vi "SPI Send Receive.vi"(7 "Chip Select DIO Pin":u8, 8 "Error In":errorcluster, 9 "Word Size (Bytes)":u8, 10 "SPI Data":u8[](array[numeric]), 11 "Arduino Resource":T1={"COM Port"="COM4", "Board Type"=enum."ChipKit uC32", "Connection Type"=enum."USB / Serial", "Baud Rate (115200)"=15, "Bytes Per Packet (15)"=15}) -> (0 "Error Out":errorcluster, 2 "SPI Data":u8[](array[numeric]), 3 "Arduino Resource":T1={"COM Port"="COM4", "Board Type"=enum."ChipKit uC32", "Connection Type"=enum."USB / Serial", "Baud Rate (115200)"=15, "Bytes Per Packet (15)"=15})   [LabVIEW 2011, in "LabVIEW Interface for ChipKit.lvlib"]
doc: "Send / Receive data bytes on the SPI bus. You must initialize the bus before you can use this VI to send / receive data."
uses:
  LabVIEW Interface for ChipKit.lvlib
  Private/Type Defs/Chipkit Resource.ctl
  Private/Type Defs/Board Type.ctl
  Private/Type Defs/Connection Type.ctl
  Private/Type Defs/Command.ctl
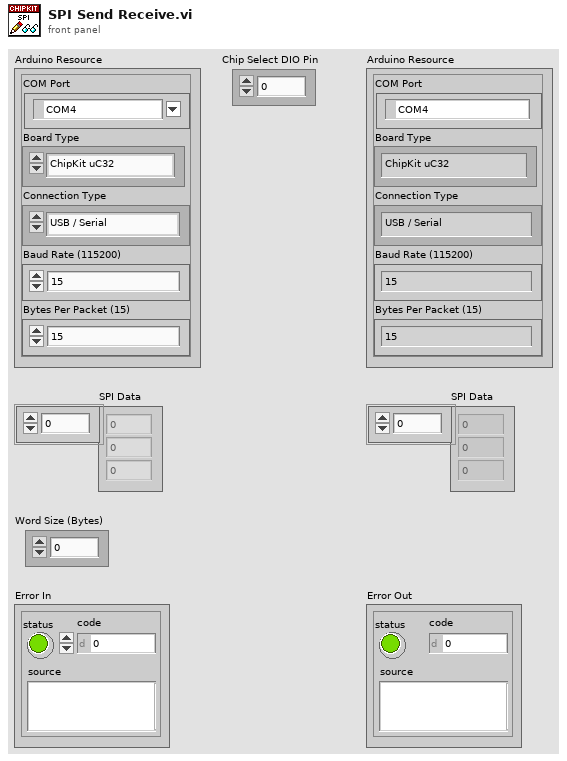
[diagram p1: front panel]
types:
  T1 = typedef "LabVIEW Interface for ChipKit.lvlib/Chipkit Resource.ctl" = cluster{"COM Port":refnum<visa-resource-name>, "Board Type":T2, "Connection Type":T3, "Baud Rate (115200)":u32, "Bytes Per Packet (15)":u32}
  T2 = typedef "LabVIEW Interface for ChipKit.lvlib/Board Type.ctl" = enum16{"ChipKit uC32", "ChipKit Uno32", "ChipKit Max32"}
  T3 = typedef "LabVIEW Interface for ChipKit.lvlib/Connection Type.ctl" = enum8{"USB / Serial", "XBEE", "BlueSmirf (Bluetooth)"}
  T4 = typedef "LabVIEW Interface for ChipKit.lvlib/Command.ctl" = enum8{"setArduinoMode", "flushSerial", "setPinMode", "digitalWritePin", "digitalWritePort", "tone", "digitalReadPin", "digitalReadPort", "analogReadPin", "analogReadPort", "pwmWritePin", "pwmWritePort", "sevenSegment_Configure", "sevenSegment_Write", "I2C Init", "I2C Write", "I2C Read", "SPI Init", "SPI Set Bit Order", "SPI Set Clock Divider", "SPI Set Data Mode", "SPI Send / Receive", "SPI Close", "Servo Set Num Servos", "Servo Config Servo", "Servo Write Angle", "Servo Read Angle", "Servo Write Pulse Width", "Servo Read Pulse Width", "Servo Detach", "LCD Init", "LCD Set Size", "LCD Set Cursor Mode", "LCD Clear", "LCD Set Cursor Position", "LCD Print", "LCD Display Power", "LCD Scroll Display", "LCD Autoscroll", "LCD Print Direction", "LCD Create Custom Char", "LCD Print Custom Char", "contAcqOn", "contAcqOff", "getFirmwareVersion", "FiniteSampleStart"}
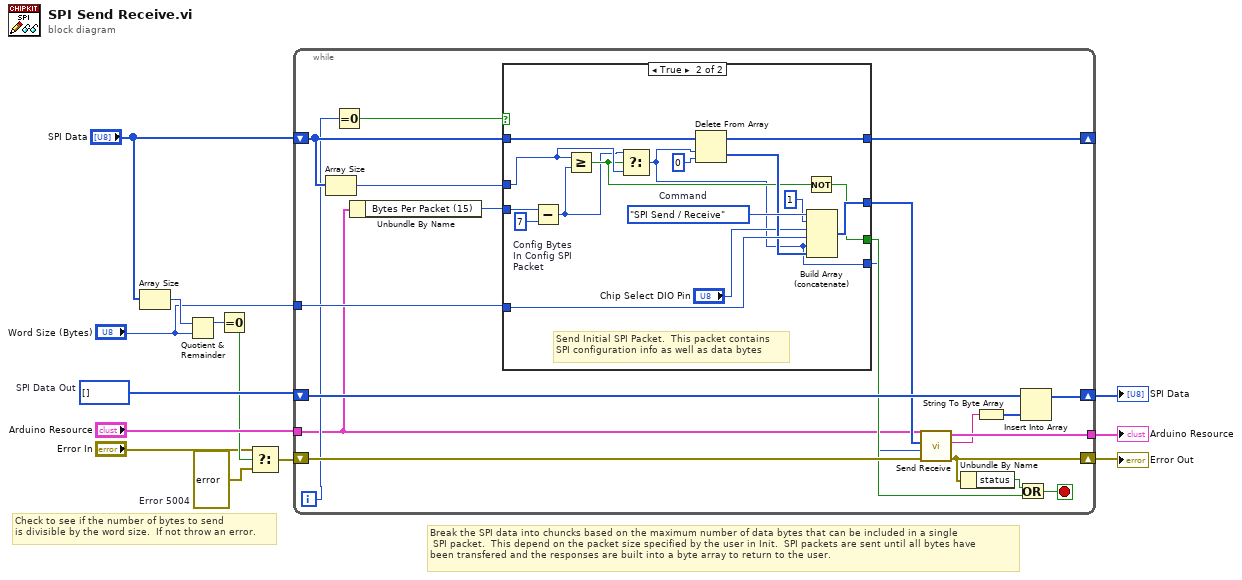
[diagram p0: block diagram]
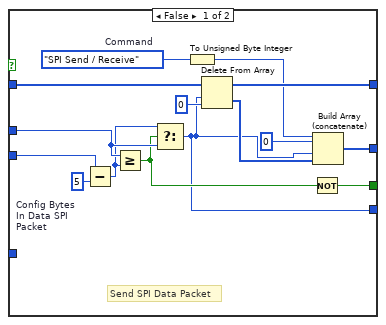
[diagram p2: hidden frame]
diagram:
  w8 = errorcluster {"status"=TRUE, "code"=5004, "source"="SPI Send Receive.  The word size is invalid for the number of SPI bytes to be sent.  The number of SPI bytes to send must be divisible by the SPI word size."}  # Error 5004
  w10 = u8[] []  # SPI Data Out
  # "Check to see if the number of bytes to send\nis divisible by the word size.  If not throw an error."
  # "Break the SPI data into chuncks based on the maximum number of data bytes that can be included in a single\n SPI packet.  This depend on the packet size specified by the user in Init.  SPI packets are sent until all bytes have \nbeen transfered and the responses are built into a byte array to return to the user."
  n1 = Array Size(array="SPI Data") -> (size(s)=w4:i32)
  n2 = Quotient & Remainder(x=w4, y="Word Size (Bytes)") -> (x-y*floor(x/y)=w7:i32)  [unwired: 1 out]
  n3 = Equal To 0?(x=w7) -> (x = 0?=w9:bool)
  n4 = Select(t="Error In", s=w9, f=w8) -> (s? t:f=w5:errorcluster)
  n5 = while {
    tunnel: "Arduino Resource" -> [w15]
    tunnel: [w33] -> w11
    shift-right: [w20] -> _
    shift-left: "SPI Data" -> [w21]
    shift-right: [w32] -> w12
    shift-left: w5 -> [w25]
    shift-right: [w27] -> w2
    shift-left: w10 -> [w28]
    tunnel: "Word Size (Bytes)" -> [w24]
    i -> [w16]
    stop <- w30 stop-if-true
    n6 = Array Size(array=w21) -> (size(s)=w23:i32)
    n7 = Equal To 0?(x=w16) -> (x = 0?=w17:bool)
    n8 = Unbundle By Name(w15) -> ("Bytes Per Packet (15)"=w14:u32)
    n9 = case shown="True" w17 {
      tunnel: [w43 w64] -> w22
      tunnel: w24 -> [_ w61]
      tunnel: w23 -> [w44 w56]
      tunnel: w21 -> [w47 w60]
      tunnel: [w46 w59] -> w20
      tunnel: [w41 w55] -> w19
      tunnel: [w37 w52] -> w18
      tunnel: w14 -> [w35 w50]
      frame False {
        w34 = u8 5  # Config Bytes In Data SPI Packet
        w40 = Command."SPI Send / Receive"  # Command
        # "Send SPI Data Packet"
        n10 = Subtract(x=w35, y=w34) -> (x-y=w36:u32)
        n11 = Greater Or Equal?(x=w44, y=w36) -> (x >= y?=w42:bool)
        n12 = Select(t=w36, s=w42, f=w44) -> (s? t:f=w37:u32)
        n13 = To Unsigned Byte Integer(number=w40) -> (unsigned 8bit integer=w39:u8)
        n14 = Delete From Array(array=w47, length=w37, index=0) -> (deleted portion=w38:u8[], array with subset deleted=w46:u8[])
        n15 = Not(x=w42) -> (.not. x?=w41:bool)
        n16 = Build Array (concatenate)(w39, u8 0 ("Bytes To Read (0)"), w37, w38) -> (w43:u32[])
      }
      frame True {
        w51 = u8 7  # Config Bytes In Config SPI Packet
        w63 = Command."SPI Send / Receive"  # Command
        # "Send Initial SPI Packet.  This packet contains\nSPI configuration info as well as data bytes"
        n17 = Subtract(x=w50, y=w51) -> (x-y=w49:u32)
        n18 = Greater Or Equal?(x=w56, y=w49) -> (x >= y?=w54:bool)
        n19 = Select(t=w49, s=w54, f=w56) -> (s? t:f=w52:u32)
        n20 = Delete From Array(array=w60, length=w52, index=0) -> (deleted portion=w58:u8[], array with subset deleted=w59:u8[])
        n21 = Not(x=w54) -> (.not. x?=w55:bool)
        n22 = Build Array (concatenate)(w63, u8 1 ("Bytes To Read (0)"), "Chip Select DIO Pin", w61, w52, w58) -> (w64:u32[])
      }
    }
    n23 = call "Send Receive.vi"("Error In"=w25, "Bytes To Read (0)"=w18, "Data"=w22, "ChipKit Resource"=w15) -> ("Error Out"=w32:errorcluster, "Read Buffer"=w29:string, "ChipKit Resource"=w33:T1)  [unwired: 5 in]
    n24 = Unbundle By Name(w32) -> ("status"=w31:bool)
    n25 = String To Byte Array(string=w29) -> (unsigned byte array=w26:u8[])
    n26 = Or(x=w31, y=w19) -> (x .or. y?=w30:bool)
    n27 = Insert Into Array(array=w28, new element=w26) -> (w27:u8[])  [unwired: 1 in]
  }
  "Error Out" <- w12
  "Arduino Resource" <- w11
  "SPI Data" <- w2
